vi "subAcquisition_MC3DInfo.vi"(0 "TI-Ctrl":T3={"Obj"=6, "Cube Bottom"=1, "Cube Top"=4, "PFS-Ctrl"={"PFS IO"=FALSE, "PSF Err"=FALSE, "PSF Pos"=0}, "Z-Ctrl"={"Z-pos"=499.75, "Home"=TRUE, "Sensitivity"=1}, "Condenser"=2, "Lightpath"=enum."EYE"} {"Condenser" items=["A"=1, "DICN2"=2, "- empty 3 -"=3, "- empty 4 -"=4, "- empty 5 -"=5, "- empty 6 -"=6]; "Z-Ctrl"."Sensitivity" min=1 max=3 step=1 scale=1.0..3.0; "PFS-Ctrl"."PSF Pos" scale=0.0..16400.0; "Cube Top" items=["Cy5"=1, "TxRed"=2, "mO2"=3, "GFP-B"=4, "DAPI"=5, "- empty 6 -"=6]; "Cube Bottom" items=["- empty 1 -"=1, "- empty 2 -"=2, "- empty 3 -"=3, "- empty 4 -"=4, "- empty 5 -"=5, "- empty 6 -"=6]; "Obj" items=["20x/.75 Dry PFS"=1, " 40x/1.3 Oil PFS"=2, "60x/1.4 Oil PFS"=3, "- empty 4 -"=4, "- empty 5 -"=5, "- empty 6 -"=6]}, 1 "ROI":T1={"Bin"=1, "ROI"={"x offset"=0, "y offset"=0, "x width"=2048, "y width"=2048}} {"ROI"."x offset" min=1 max=512 step=1; "ROI"."y offset" min=1 max=512 step=1; "ROI"."x width" min=1 max=512 step=1; "ROI"."y width" min=1 max=512 step=1; "Bin" items=["1x1"=1, "2x2"=2, "4x4"=4]}, 2 "Camera in use":T2={"Model"="-", "Camera ID"="-", "Bits"=0}, 5 "FWPosition":i32, 9 "DO":T4, 11 "AO (V)":dbl[](array[numeric])=[0.0, 0.0, 0.0, 0.0, 0.0] min=0.0 max=5.0 step=0.01, 12 "Exposure (msec)":dbl=100.0 min=1.0 max=5000.0 step=1.0, 13 "Positions":dbl[](array[numeric])=[55.78, 33.02, 0.0]) -> (8 "Text":string="nrow = \t240\rncol = \t192\rrow offset = \t896\rcol offset = \t784\rBinning =\t1\r============== \r594nm eff. =\t1.000000\r Exposure (msec) =\t0\r------------- \r488 weak eff. =\t0.000000\r Exposure (msec) =\t1\r------------- \rEmission filter =\tET575/50\r============== ")   [LabVIEW 2015]
panel:
  # "LED"
  # "637"
  # "561"
  # "532"
  # "488"
  # "405"
  # "Global"
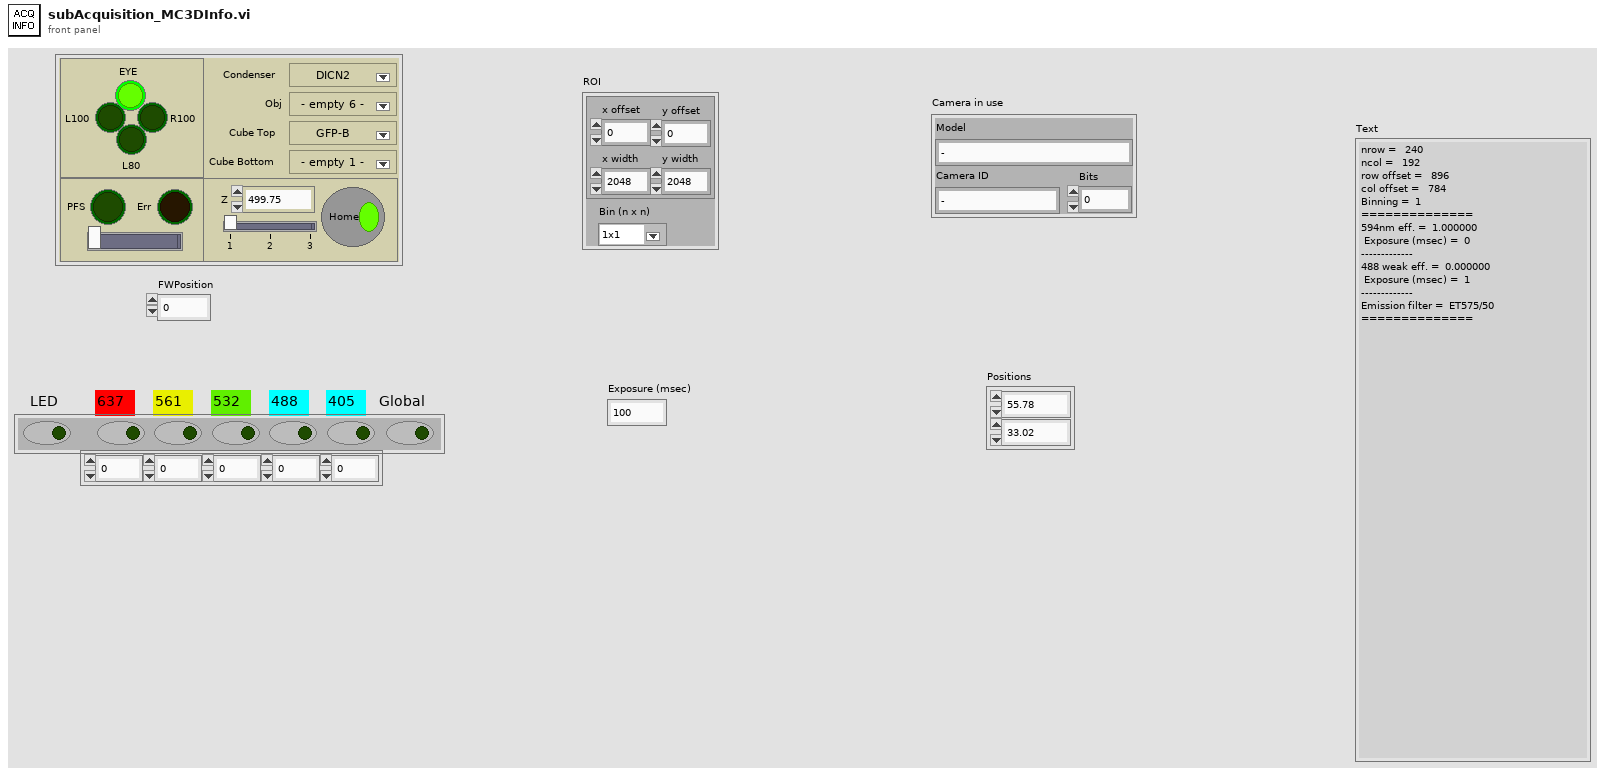
[diagram p1: front panel]
types:
  T1 = cluster{"Bin":u16, "ROI":cluster{"x offset":i32, "y offset":i32, "x width":i32, "y width":i32}}
  T2 = cluster{"Model":string, "Camera ID":string, "Bits":i32}
  T3 = cluster{"Obj":u16, "Cube Bottom":u16, "Cube Top":u16, "PFS-Ctrl":cluster{"PFS IO":bool, "PSF Err":bool, "PSF Pos":u32}, "Z-Ctrl":cluster{"Z-pos":dbl, "Home":bool, "Sensitivity":u8}, "Condenser":u16, "Lightpath":enum32{"EYE", "L100", "R100", "L80"}}
  T4 = cluster{"DO 1":bool, "DO 2":bool, "DO 3":bool, "DO 4":bool, "DO 5":bool, "LED":bool, "Global":bool}
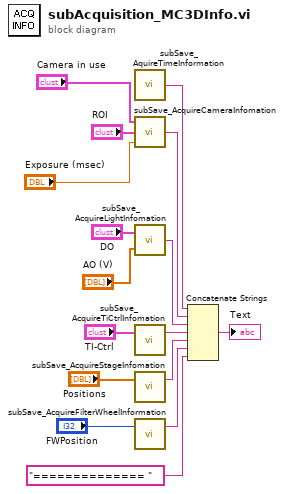
[diagram p0: block diagram]
diagram:
  n1 = call "subSave_AquireTimeInformation.vi"() -> ("time out"=w14:string)  [unwired: 1 in]
  n2 = call "subSave_AcquireCameraInfomation.vi"("Exposure (msec)"="Exposure (msec)", "ROI"="ROI", "Camera in use"="Camera in use") -> ("Text Out"=w2:string)
  n3 = call "subSave_AcquireLightInfomation.vi"("AO (V)"="AO (V)", "DO"="DO") -> ("Text out"=w11:string)
  n4 = call "subSave_AcquireTiCtrlInfomation.vi"("TI-Ctrl"="TI-Ctrl") -> ("Text out"=w9:string)  [unwired: 2 in]
  n5 = call "subSave_AcquireStageInfomation.vi"("Positions"="Positions") -> ("Text out"=w7:string)  [unwired: 2 in]
  n6 = call "subSave_AcquireFilterWheelInformation.vi"("FWPosition"="FWPosition") -> ("FW text"=w6:string)  [unwired: 2 in]
  n7 = Concatenate Strings(w14, w2, w11, w9, w7, w6, "============== " ("string")) -> (→"Text":string)
